vi "Filter_ChA(SubVI).vi"(9 "sample length":i32=100, 10 "input":dbl, 11 "Filter on":bool) -> (2 "Output Number":dbl, 3 "Output":cluster{"Frequency Interpolate / Hz":dbl}(graph))   [LabVIEW 2015]
uses:
  <vilib>/ptbypt/NI_PtbyPt.lvlib
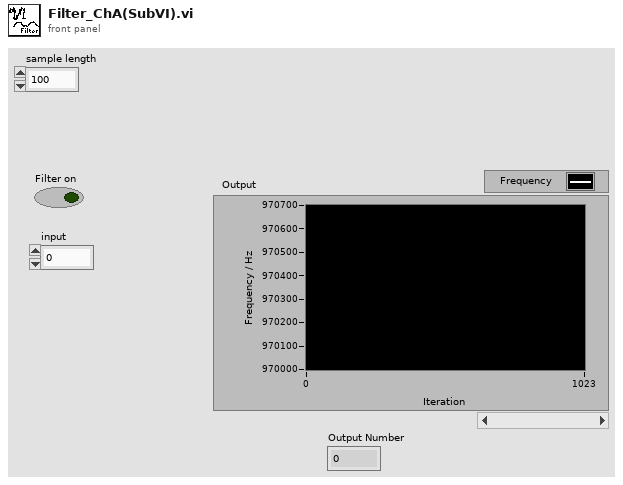
[diagram p1: front panel]
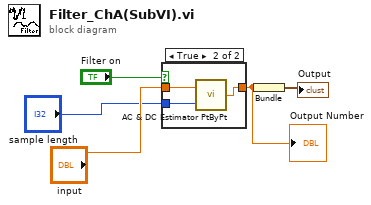
[diagram p0: block diagram]
diagram:
  n1 = case shown="True" "Filter on" {
    tunnel: "input" -> [w6 w9]
    tunnel: [w6 w8] -> w2
    tunnel: "sample length" -> [_ w7]
    frame False {
    }
    frame True {
      n2 = call <vilib>:"AC & DC Estimator PtByPt.vi"("signal"=w9, "sample length"=w7) -> ("DC estimate (V)"=w8:dbl)  [unwired: 1 in, 2 out]
    }
  }
  "Output Number" <- w2
  n3 = Bundle("DC estimate (V)"=w2) -> (→"Output":cluster{"DC estimate (V)":dbl})  [unwired: 1 in]
